vi "get_all_qcm_life.vi"(8 "error in (no error)":errorcluster, 11 "VISA resource name":refnum<visa-resource-name>) -> (0 "error out":errorcluster, 2 "Life array (%)":u8[](array[numeric]), 3 "VISA resource name out":refnum<visa-resource-name>)   [LabVIEW 2018, in "Inficon IC6.lvlib"]
doc: "Query the percentage life remaining of all crystal monitors."
uses:
  <instrlib>/Inficon IC6/Inficon IC6.lvlib
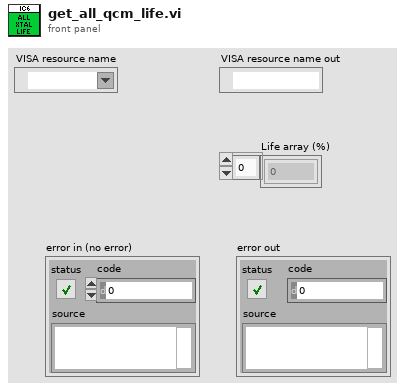
[diagram p1: front panel]
types:
  T1 = enum16{"Source", "General", "Input name", "Process name", "Logic", "Material", "Material name", "Output name", "Process", "Sensor", "Output type", "User message", "Layer", ""}
  T2 = enum16{"Hello", "Query", "Remote action", "Status", "Update"}
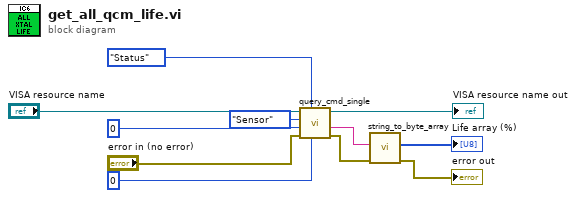
[diagram p0: block diagram]
diagram:
  n1 = call <instrlib>:"query_cmd_single.vi"("Parameter"=u8 0 ("Sensor"), "Command group"=T2."Status", "error in (no error)"="error in (no error)", "Command ID"=u8 0, "Command subgroup"=T1."Sensor", "VISA resource name"="VISA resource name") -> ("error out"=w4:errorcluster, "formatted response"=w2:string, "VISA resource name out"=→"VISA resource name out":refnum<visa-resource-name>)  [unwired: 1 in, 2 out]
  n2 = call <instrlib>:"string_to_byte_array.vi"("error in (no error)"=w4, "Byte"=w2) -> ("error out"=→"error out":errorcluster, "Int array"=→"Life array (%)":u8[])  [unwired: 8 in]
